vi "parser_test_01.vi"() -> ()   [LabVIEW 2010]
panel:
  in  "String 2":string
  out "Array 2":string[](array[string])
  out "size(s)":i32
  out "Array":string[](array[string])
  in  "String":string
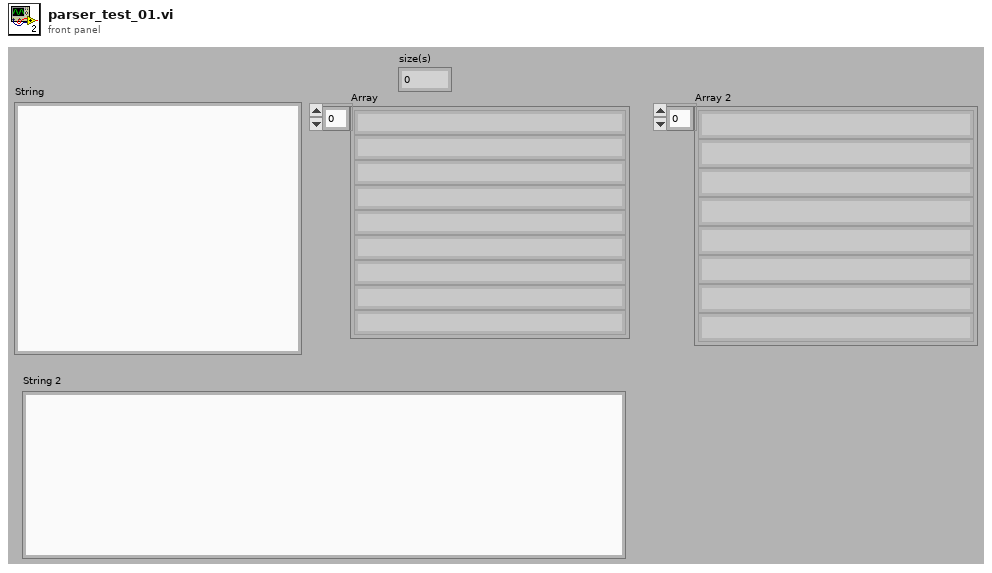
[diagram p1: front panel]
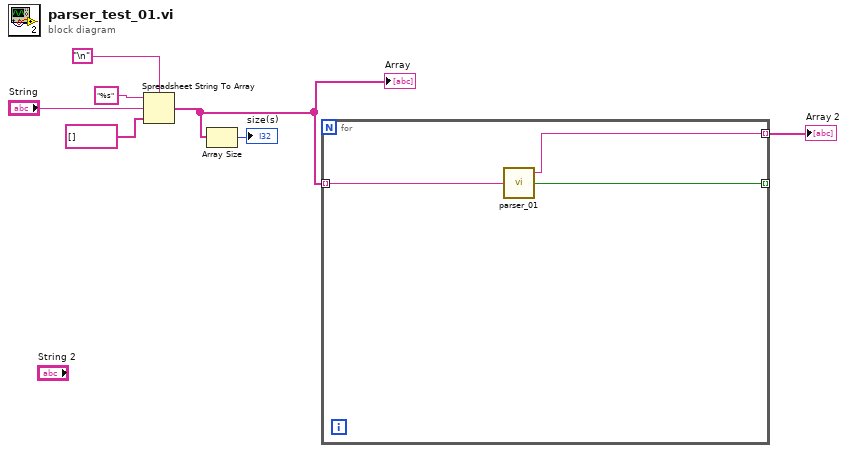
[diagram p0: block diagram]
diagram:
  n1 = Spreadsheet String To Array(delimiter (Tab)="\n", format string="%s", spreadsheet string="String", array type (2D Dbl)=string[] []) -> (array=w4:string[])
  "Array" <- w4
  n2 = Array Size(array=w4) -> (size(s)=→"size(s)":i32)
  n3 = for {
    tunnel: w4 -> [w10] mode=indexing
    tunnel: [w9] -> _ mode=indexing
    tunnel: [w8] -> w1 mode=indexing
    n4 = call "parser_01.vi"("data in"=w10) -> ("Exit"=w9:bool, "Answer"=w8:string)  [unwired: 3 in]
  }
  "Array 2" <- w1
